vi "Configure Temperature (Thermistor).vi"(0 "VISA resource name":refnum<visa-resource-name>, 1 "Unit (1: Celsius)":i32(ring)=1 items=["Kelvin", "Celsius", "Fahrenheit"], 5 "Thermistor Type (1: 5000)":i32(ring)=1 items=["2252", "5000", "10000"], 9 "Channel List(\"\")":string, 11 "error in (no error)":errorcluster) -> (4 "VISA resource name out":refnum<visa-resource-name>, 15 "error out":errorcluster)   [LabVIEW 2019, in "Keithley DMM6500 DAQ6500 Series.lvlib"]
doc: "Configures temperature measurement with thermistor."
uses:
  Keithley DMM6500 DAQ6500 Series.lvlib
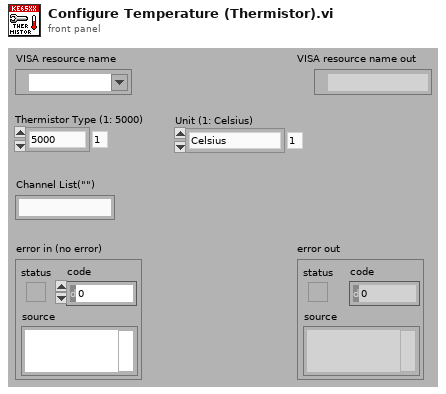
[diagram p1: front panel]
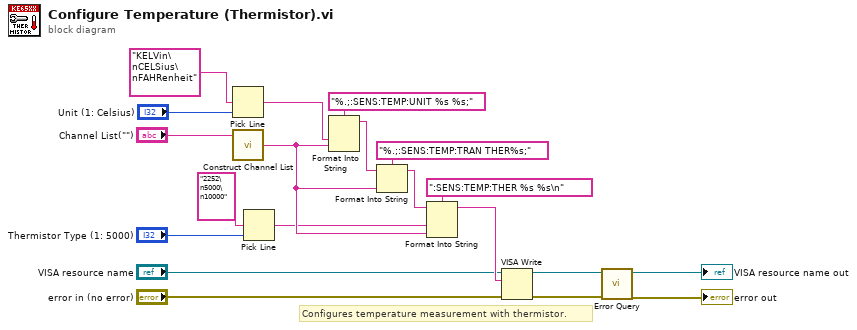
[diagram p0: block diagram]
diagram:
  # "Configures temperature measurement with thermistor."
  n1 = Pick Line(multi-line string="KELVin\nCELSius\nFAHRenheit", line index="Unit (1: Celsius)") -> (output string=w8:string)  [unwired: 1 in]
  n2 = call "Construct Channel List.vi"("Channel List"="Channel List(\"\")") -> ("Channel List String"=w5:string)  [unwired: 2 in]
  n3 = Pick Line(multi-line string="2252\n5000\n10000", line index="Thermistor Type (1: 5000)") -> (output string=w3:string)  [unwired: 1 in]
  n4 = Format Into String(format string="%.;:SENS:TEMP:UNIT %s %s;", w8, w5) -> (resulting string=w2:string)  [unwired: 2 in, 1 out]
  n5 = Format Into String(format string="%.;:SENS:TEMP:TRAN THER%s;", initial string=w2, w5) -> (resulting string=w19:string)  [unwired: 1 in, 1 out]
  n6 = Format Into String(format string=":SENS:TEMP:THER %s %s\n", initial string=w19, w3, w5) -> (resulting string=w17:string)  [unwired: 1 in, 1 out]
  n7 = VISA Write(VISA resource name="VISA resource name", write buffer=w17, error in (no error)="error in (no error)") -> (VISA resource name out=w14:refnum<visa-resource-name>, error out=w13:errorcluster)  [unwired: 1 out]
  n8 = call "Error Query.vi"("error in (no error)"=w13, "VISA resource name"=w14) -> ("error out"=→"error out":errorcluster, "VISA resource name out"=→"VISA resource name out":refnum<visa-resource-name>)  [unwired: 6 in, 2 out]
